vi "RIO.vi"() -> ()   [LabVIEW 2015]
uses:
  <vilib>/rvi/interface/nirviOpenFPGA/nirviOpenFPGA.xnode
  <vilib>/rvi/interface/nirviMethod/nirviMethod.xnode
  <vilib>/FPGAPlugInAG/Dynamic/niLvFpga_Abort_Dynamic.vi
  <vilib>/FPGAPlugInAG/Dynamic/niLvFpga_Run_Dynamic.vi
  <vilib>/FPGAPlugInAG/Dynamic/niLvFpga_ReadFifo_Dynamic.vi
  <vilib>/rvi/errors/niLvFpgaMergeErrorWithErrorCode.vi
  <vilib>/NI_Real-Time Target Support.lvlib
  rio_Global.vi
  FPGA Bitfiles/autonomous_FPGATarget4_fpga1_rudp+OsNkSQ.lvbitx
  samsung/fpga 1.vi
  <vilib>/FPGAPlugInAG/cRIO-9030/niLvFpga_Open_cRIO-9030.vi
  <vilib>/rvi/interface/common/dynamic/niFpgaDynamicAddResources.vi
panel:
  out "status":string
  out "PRND":string
  out "left light":bool
  out "right light":bool
  out "Speed2":i16 format="%02.0f"
  out "SPEED":dbl(knob) scale=0.0..200.0 scale format="%_2p"
  out "tic":u32
  out "filesave":refnum<file>
  out "FPGA":refnum<k20>
  out "APV":u8(slide) scale=0.0..100.0
  out "brake":u8(slide) scale=0.0..100.0
  # "km/h"
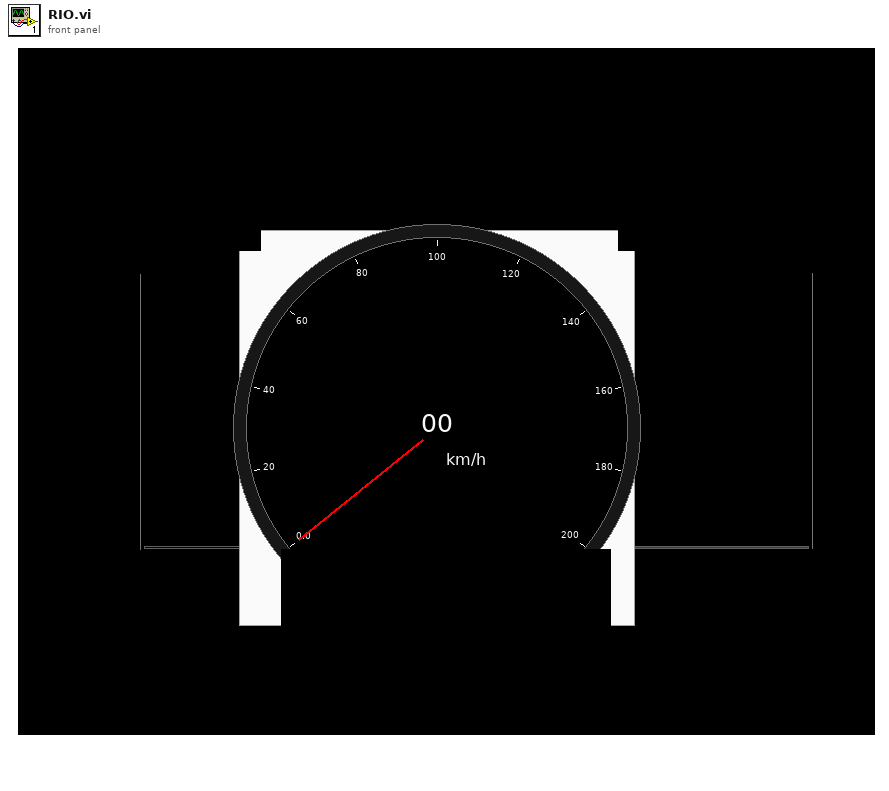
[diagram p1: front panel]
types:
  T1 = enum16{"open", "replace", "create", "open or create", "replace or create", "replace or create with confirmation"}
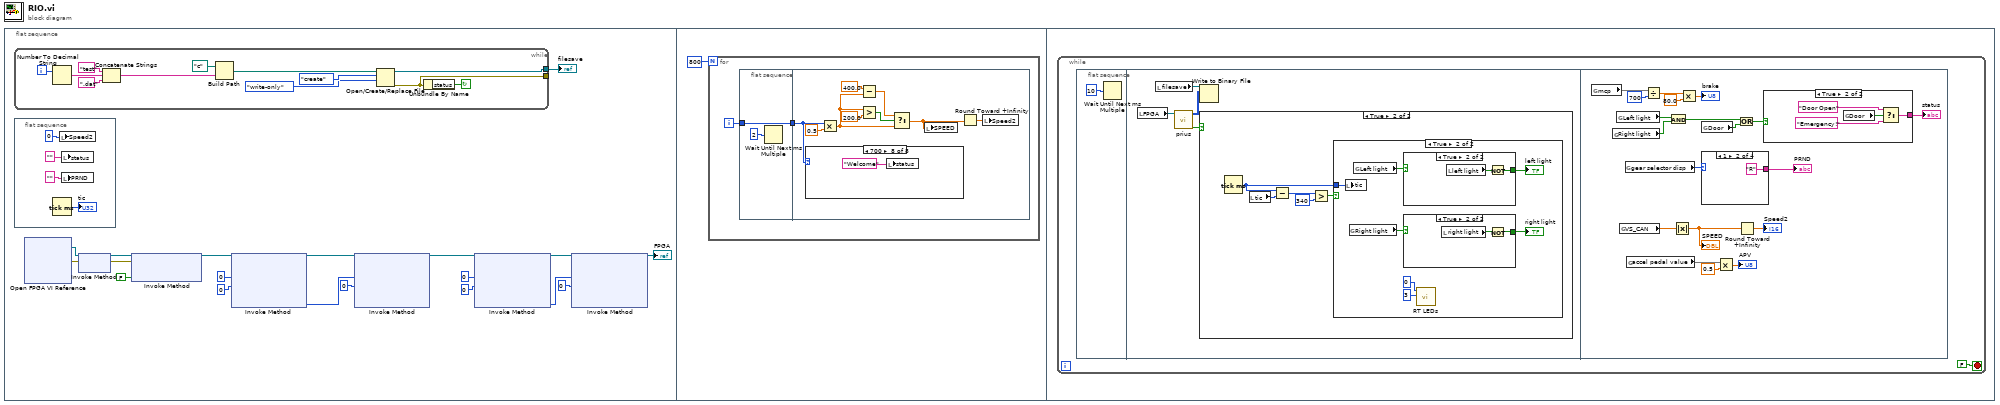
[diagram p0: block diagram]
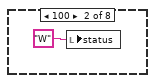
[diagram p3: hidden frame]
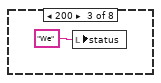
[diagram p4: hidden frame]
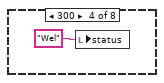
[diagram p5: hidden frame]
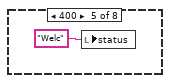
[diagram p6: hidden frame]
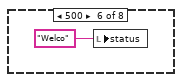
[diagram p7: hidden frame]
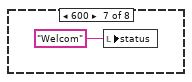
[diagram p8: hidden frame]
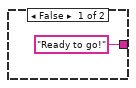
[diagram p13: hidden frame]
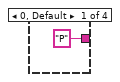
[diagram p14: hidden frame]
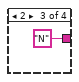
[diagram p15: hidden frame]
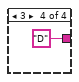
[diagram p16: hidden frame]
diagram:
  n1 = flat-sequence {
    frame #0 {
      n2 = while {
        tunnel: [w34] -> w1
        tunnel: [w25] -> _
        i -> [w31]
        stop <- w24 continue-if-true
        n3 = Number To Decimal String(number=w31) -> (decimal integer string=w29:string)  [unwired: 1 in]
        n4 = Concatenate Strings("test" ("string"), w29, ".dat" ("string")) -> (w27:string)
        n5 = Build Path(base path=path "c:/" ("file path (use dialog)"), name or relative path=w27) -> (appended path=w30:path)
        n6 = Open/Create/Replace File(file path (use dialog)=w30, operation (0:open)=T1."create", access (0:read/write)=enum16{"read/write", "read-only", "write-only"}."write-only") -> (refnum out=w34:refnum<file>, error out=w25:errorcluster)  [unwired: 3 in, 1 out]
        n7 = Unbundle By Name(w25) -> ("status"=w24:bool)
      }
      "filesave" <- w1
      n8 = flat-sequence {
        frame #0 {
          n9 = Tick Count (ms)() -> (millisecond timer value=→"tic":u32)
          n10 = local write "Speed2"(i16 0 ("Speed2")) -> ()
          n11 = local write "status"("" ("status")) -> ()
          n12 = local write "PRND"("" ("PRND")) -> ()
        }
      }
      n13 = xnode "Open FPGA VI Reference"() -> ("FPGA VI Reference Out"=w19:refnum<k20>, "error out"=w18:errorcluster)  [unwired: 2 in]
      n14 = xnode "Invoke Method"("FPGA VI Reference In"=w19, "error in"=w18) -> ("FPGA VI Reference Out"=w17:refnum<k20>, "error out"=w16:errorcluster)
      n15 = xnode "Invoke Method"("FPGA VI Reference In"=w17, "error in"=w16, "Wait Until Done (F)"=FALSE) -> ("FPGA VI Reference Out"=w14:refnum<k20>)  [unwired: 1 out]
      n16 = xnode "Invoke Method"("FPGA VI Reference In"=w14, "Number of Elements"=u32 0, "Timeout (ms)"=0) -> ("FPGA VI Reference Out"=w12:refnum<k20>, "Elements Remaining"=w11:u32)  [unwired: 1 in, 2 out]
      n17 = xnode "Invoke Method"("FPGA VI Reference In"=w12, "Number of Elements"=w11, "Timeout (ms)"=0) -> ("FPGA VI Reference Out"=w7:refnum<k20>)  [unwired: 1 in, 3 out]
      n18 = xnode "Invoke Method"("FPGA VI Reference In"=w7, "Number of Elements"=u32 0, "Timeout (ms)"=0) -> ("FPGA VI Reference Out"=w9:refnum<k20>, "Elements Remaining"=w10:u32)  [unwired: 1 in, 2 out]
      n19 = xnode "Invoke Method"("FPGA VI Reference In"=w9, "Number of Elements"=w10, "Timeout (ms)"=0) -> ("FPGA VI Reference Out"=→"FPGA":refnum<k20>)  [unwired: 1 in, 3 out]
    }
    frame #1 {
      n20 = for {
        N: 800 -> [_]
        i -> [w37]
        n21 = flat-sequence {
          tunnel: [w39] -> w38
          tunnel: w37 -> [w39]
          tunnel: w38 -> [w41]
          frame #0 {
            n22 = Wait Until Next ms Multiple(millisecond multiple=u32 2) -> ()  [unwired: 1 out]
          }
          frame #1 {
            n23 = case shown="700" w41 {
              frame 0, Default {
              }
              frame 100 {
                n24 = local write "status"("W" ("status")) -> ()
              }
              frame 200 {
                n25 = local write "status"("We" ("status")) -> ()
              }
              frame 300 {
                n26 = local write "status"("Wel" ("status")) -> ()
              }
              frame 400 {
                n27 = local write "status"("Welc" ("status")) -> ()
              }
              frame 500 {
                n28 = local write "status"("Welco" ("status")) -> ()
              }
              frame 600 {
                n29 = local write "status"("Welcom" ("status")) -> ()
              }
              frame 700 {
                n30 = local write "status"("Welcome" ("status")) -> ()
              }
            }
            n31 = Multiply(x=w41, y=0.5) -> (x*y=w44:dbl)
            n32 = Subtract(x=400.0, y=w44) -> (x-y=w45:dbl)
            n33 = Greater?(x=w44, y=200.0) -> (0:w47:bool)
            n34 = Select(t=w45, s=w47, f=w44) -> (s? t:f=w43:dbl)
            n35 = local write "SPEED"(w43) -> ()
            n36 = Round Toward +Infinity(x=w43) -> (ceil(x): smallest int >= x=w42:dbl)
            n37 = local write "Speed2"(w42) -> ()
          }
        }
      }
    }
    frame #2 {
      n38 = while {
        stop <- FALSE stop-if-true
        n39 = flat-sequence {
          frame #0 {
            n40 = Wait Until Next ms Multiple(millisecond multiple=u32 10) -> ()  [unwired: 1 out]
          }
          frame #1 {
            n41 = local read "FPGA"() -> (w61:refnum<k20>)
            n42 = local read "filesave"() -> (w62:refnum<file>)
            n43 = call "prius.vi"("FPGA"=w61) -> ("can enabled"=w59:bool, "CAN Data"=w60:u8[][])  [unwired: 9 in]
            n44 = Write to Binary File(file (use dialog)=w62, data=w60) -> ()  [unwired: 4 in, 3 out]
            n45 = case shown="True" w59 {
              frame False {
              }
              frame True {
                n46 = Tick Count (ms)() -> (millisecond timer value=w66:u32)
                n47 = local read "tic"() -> (w63:u32)
                n48 = Subtract(x=w66, y=w63) -> (x-y=w64:u32)
                n49 = Greater?(x=w64, y=u32 340) -> (0:w67:bool)
                n50 = case shown="True" w67 {
                  tunnel: w66 -> [_ w74]
                  frame False {
                  }
                  frame True {
                    n51 = local write "tic"(w74) -> ()
                    n52 = global read "rio_Global.vi" "Right light"() -> (w69:bool)
                    n53 = global read "rio_Global.vi" "Left light"() -> (w71:bool)
                    n54 = case shown="True" w71 {
                      tunnel: [_ w77] -> w70
                      frame False {
                      }
                      frame True {
                        n55 = local read "left light"() -> (w78:bool)
                        n56 = Not(x=w78) -> (.not. x?=w77:bool)
                      }
                    }
                    "left light" <- w70
                    n57 = case shown="True" w69 {
                      tunnel: [_ w75] -> w68
                      frame False {
                      }
                      frame True {
                        n58 = local read "right light"() -> (w76:bool)
                        n59 = Not(x=w76) -> (.not. x?=w75:bool)
                      }
                    }
                    "right light" <- w68
                    n60 = call <vilib>:"RT LEDs.vi"("State"=3, "LED Num"=0) -> ()  [unwired: 4 in, 2 out]
                  }
                }
              }
            }
          }
          frame #2 {
            n61 = global read "rio_Global.vi" "mcp"() -> (w86)
            n62 = global read "rio_Global.vi" "Right light"() -> (w91:bool)
            n63 = global read "rio_Global.vi" "Left light"() -> (w90:bool)
            n64 = global read "rio_Global.vi" "VS_CAN"() -> (w97:dbl)
            n65 = global read "rio_Global.vi" "gear selector disp"() -> (w96:u8)
            n66 = global read "rio_Global.vi" "accel pedal value"() -> (w80)
            n67 = Divide(x=w86, y=u16 700) -> (x/y=w84:dbl)
            n68 = And(x=w90, y=w91) -> (x .and. y?=w89:bool)
            n69 = Absolute Value(x=w97) -> (abs(x)=w94:dbl)
            "SPEED" <- w94
            n70 = Multiply(x=w84, y=80.0) -> (x*y=→"brake":dbl)
            n71 = global read "rio_Global.vi" "Door"() -> (w88:bool)
            n72 = case shown="1" w96 {
              tunnel: ["P" "R" "N" "D"] -> w95
              frame 0, Default {
              }
              frame 1 {
              }
              frame 2 {
              }
              frame 3 {
              }
            }
            "PRND" <- w95
            n73 = Multiply(x=w80, y=0.5) -> (x*y=→"APV":dbl)
            n74 = Or(x=w89, y=w88) -> (x .or. y?=w87:bool)
            n75 = Round Toward +Infinity(x=w94) -> (ceil(x): smallest int >= x=→"Speed2":dbl)
            n76 = case shown="True" w87 {
              tunnel: ["Ready to go!" w100] -> w92
              frame False {
              }
              frame True {
                n77 = global read "rio_Global.vi" "Door"() -> (w102:bool)
                n78 = Select(t="Door Open", s=w102, f="Emergency!") -> (s? t:f=w100:string)
              }
            }
            "status" <- w92
          }
        }
      }
    }
  }
